vi "Multigas test.vi"() -> ()   [LabVIEW 2011]
panel:
  in  "stop":bool
  out "Array":dbl[](array[numeric])
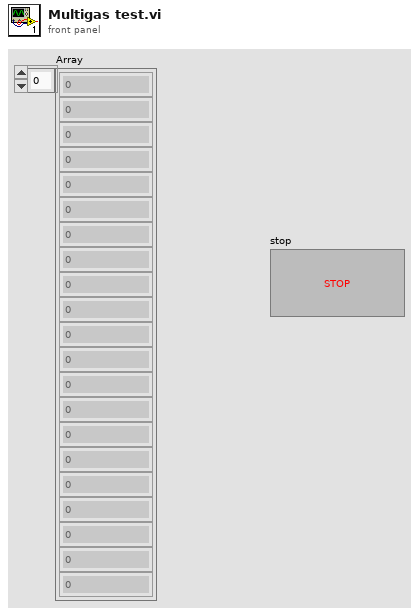
[diagram p1: front panel]
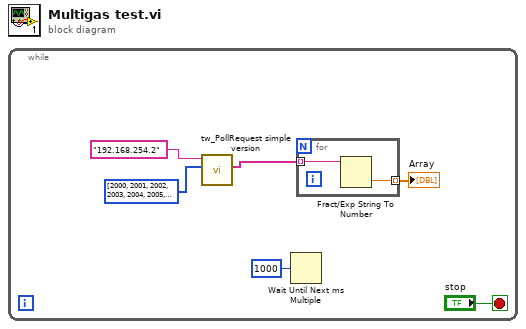
[diagram p0: block diagram]
diagram:
  n1 = while {
    stop <- "stop" stop-if-true
    n2 = call <userlib>:"tw_PollRequest simple version.vi"("EVID list"=i32[] [2000, 2001, 2002, 2003, 2004, 2005, 2006, 2007, 2008, 2009, 2010, 2011, 2012, 2013, 2014], "IP_ADD [127.0.0.1]"="192.168.254.2") -> ("values out"=w5:string[])  [unwired: 7 in, 2 out]
    n3 = Wait Until Next ms Multiple(millisecond multiple=u32 1000) -> ()  [unwired: 1 out]
    n4 = for {
      tunnel: [w8] -> w3 mode=indexing
      tunnel: w5 -> [w7] mode=indexing
      n5 = Fract/Exp String To Number(string=w7) -> (number=w8:dbl)  [unwired: 3 in, 1 out]
    }
    "Array" <- w3
  }
